vi "Rotate Flip Layer.vi"(8 "error in (no error)":errorcluster, 9 "Rotate":bool, 10 "Reset origin?":bool, 11 "Layer in":refnum<class "Layer.lvclass">) -> (0 "error out":errorcluster, 3 "Layer out":refnum<class "Layer.lvclass">)   [LabVIEW 2021, in "LabVIEW Icon API.lvlib"]
doc: "Rotate or Flip the User Layer glyph."
uses:
  LabVIEW Icon API.lvlib
  lv_icon/Classes/Layer/Layer.lvclass
  lv_icon/lv_icon.lvlib
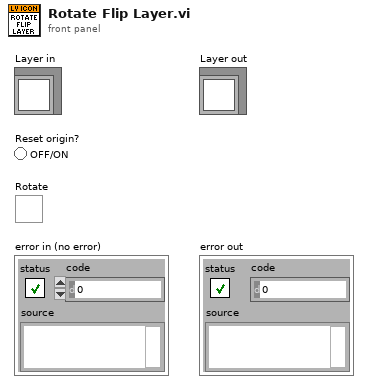
[diagram p1: front panel]
types:
  T1 = cluster{"left":i16, "top":i16, "right":i16, "bottom":i16}
  T2 = typedef "Layer.ctl" = cluster{"LayerIcon":picture, "LayerName":string, "Opacity":u8, "Visibility?":bool}
  T3 = typedef "LVPoint32TypeDef.ctl" = cluster{"Horizontal":i32, "Vertical":i32}
  T4 = cluster{"left":i16, "top":i16, "bottom":i16, "right":i16}
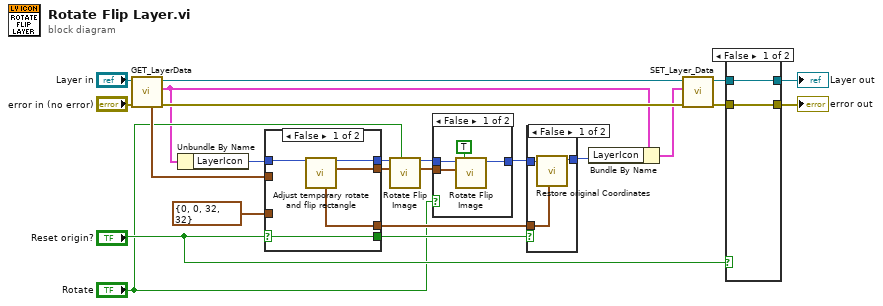
[diagram p0: block diagram]
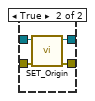
[diagram p2: hidden frame]
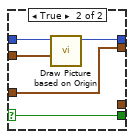
[diagram p4: hidden frame]
diagram:
  n1 = call-dynamic "GET_LayerData.vi"("error in (no error)"="error in (no error)", "Layer.lvclass in"="Layer in") -> ("error out"=w5:errorcluster, "Data"=w4:T2, "Layer.lvclass out"=w2:refnum<class "Layer.lvclass">, "Origin"=w22:T3)  [unwired: 6 out]
  n2 = Unbundle By Name(w4) -> ("LayerIcon"=w21:picture)
  n3 = case shown="False" "Reset origin?" {
    selector: "Reset origin?" -> [w24 w33]
    tunnel: w21 -> [w28 w31]
    tunnel: [w27 w30] -> w10
    tunnel: [w26 w32] -> w11
    tunnel: [w25 _] -> w14
    tunnel: [w24 w33] -> w15
    tunnel: T1 {"left"=0, "top"=0, "right"=32, "bottom"=32} ("rect") -> [_ w32]
    tunnel: w22 -> [_ w29]
    frame False {
      n4 = call "Adjust temporary rotate and flip rectangle.vi"("Pic in"=w28) -> ("temp subset rect"=w26:cluster{i32, i32, "b-a":i32, "b-a":i32}, "Pic out"=w27:picture, "true subset rect"=w25:T1)  [unwired: 8 out]
    }
    frame True {
      n5 = call "Draw Picture based on Origin.vi"("Origin"=w29, "LayerIcon in"=w31) -> ("LayerIcon out"=w30:picture)  [unwired: 1 in, 8 out]
    }
  }
  n6 = call "Rotate Flip Image.vi"("Rotate?"="Rotate", "rect"=w11, "Temp Icon In"=w10) -> ("rect out"=w9:T4, "Temp Icon Out"=w8:picture)  [unwired: 7 out]
  n7 = case shown="False" "Rotate" {
    tunnel: w8 -> [w37 w38]
    tunnel: [w36 w38] -> w12
    tunnel: w9 -> [w34 _]
    frame False {
      n8 = call "Rotate Flip Image.vi"("Rotate?"=TRUE, "rect"=w34, "Temp Icon In"=w37) -> ("Temp Icon Out"=w36:picture)  [unwired: 8 out]
    }
    frame True {
    }
  }
  n9 = case shown="False" w15 {
    tunnel: w12 -> [w41 w42]
    tunnel: [w40 w42] -> w13
    tunnel: w14 -> [w39 _]
    frame False {
      n10 = call "Restore original Coordinates.vi"("temp size in"=w39, "Pic in"=w41) -> ("Pic out"=w40:picture)  [unwired: 9 out]
    }
    frame True {
    }
  }
  n11 = Bundle By Name(cluster=w4, "LayerIcon"=w13) -> (w3:T2)
  n12 = call-dynamic "SET_Layer_Data.vi"("error in (no error)"=w5, "Data"=w3, "Layer.lvclass in"=w2) -> ("error out"=w17:errorcluster, "Layer.lvclass out"=w18:refnum<class "Layer.lvclass">)  [unwired: 1 in, 6 out]
  n13 = case shown="False" "Reset origin?" {
    tunnel: w17 -> [w44 w48]
    tunnel: w18 -> [w43 w47]
    tunnel: [w43 w46] -> w19
    tunnel: [w44 w45] -> w20
    frame False {
    }
    frame True {
      n14 = call-dynamic "SET_Origin.vi"("error in (no error)"=w48, "Layer.lvclass in"=w47) -> ("error out"=w45:errorcluster, "Layer.lvclass out"=w46:refnum<class "Layer.lvclass">)  [unwired: 8 in]
    }
  }
  "error out" <- w20
  "Layer out" <- w19
